vi "XX-DBL.vi"(8 "单位":dbl=1000000.0, 9 "下限":dbl=-90.0, 10 "上限":dbl=90.0, 11 "数值输入":dbl) -> (3 "输出":dbl)   [LabVIEW 2012]
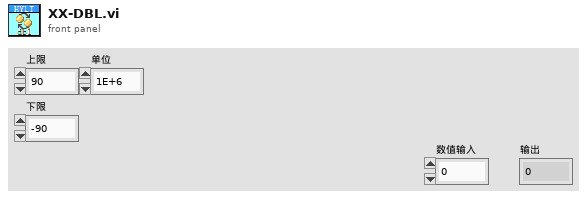
[diagram p1: front panel]
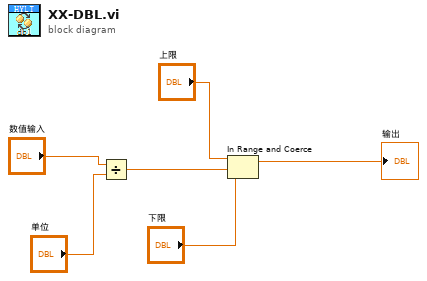
[diagram p0: block diagram]
diagram:
  n1 = Divide(x="数值输入", y="单位") -> (x/y=w6:dbl)
  n2 = In Range and Coerce(upper limit="上限", x=w6, lower limit="下限") -> (coerced(x)=→"输出":dbl)  [unwired: 1 out]
